vi "Read Arm Pot and Encoder Values.vi"(0 "error in (no error)":errorcluster) -> (1 "armPotValue":dbl, 2 "error out":errorcluster)   [LabVIEW 2019]
uses:
  Global Arm Variables.vi
  <vilib>/Rock Robotics/Network Tables/NT Write Number.vi
  <vilib>/Rock Robotics/Network Tables/NT Write Boolean.vi
panel:
  out "IllegalRangeForExtendedArm":bool
  out "armAngle(degrees)":sgl
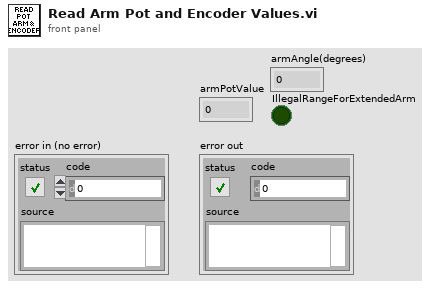
[diagram p1: front panel]
types:
  T1 = typedef "WPI_PotentiometerDevRef.ctl" = cluster{"DevStatus":errorcluster, "Analog Channel":T2, "Invert Output":bool}
  T2 = typedef "FPGA_AIChannel.ctl" = enum8{"AI 0", "AI 1", "AI 2", "AI 3", "AI MXP 0", "AI MXP 1", "AI MXP 2", "AI MXP 3", "Invalid"}
  T3 = typedef "WPI_EncoderDevRef.ctl" = cluster{"DevStatus":errorcluster, "EncoderIndex":T4, "CounterIndex":T5, "DistancePerCount":dbl, "Decoding Type":T6}
  T4 = typedef "FPGA_EncoderIdx.ctl" = enum8{"Enc 0", "Enc 1", "Enc 2", "Enc 3", "Enc 4", "Enc 5", "Enc 6", "Enc 7", "Invalid"}
  T5 = typedef "FPGA_CounterCtrSystemIndex.ctl" = enum8{"Ctr 0", "Ctr 1", "Ctr 2", "Ctr 3", "Ctr 4", "Ctr 5", "Ctr 6", "Ctr 7", "Invalid"}
  T6 = typedef "WPI_EncoderType.ctl" = enum16{"1x", "2x", "4x"}
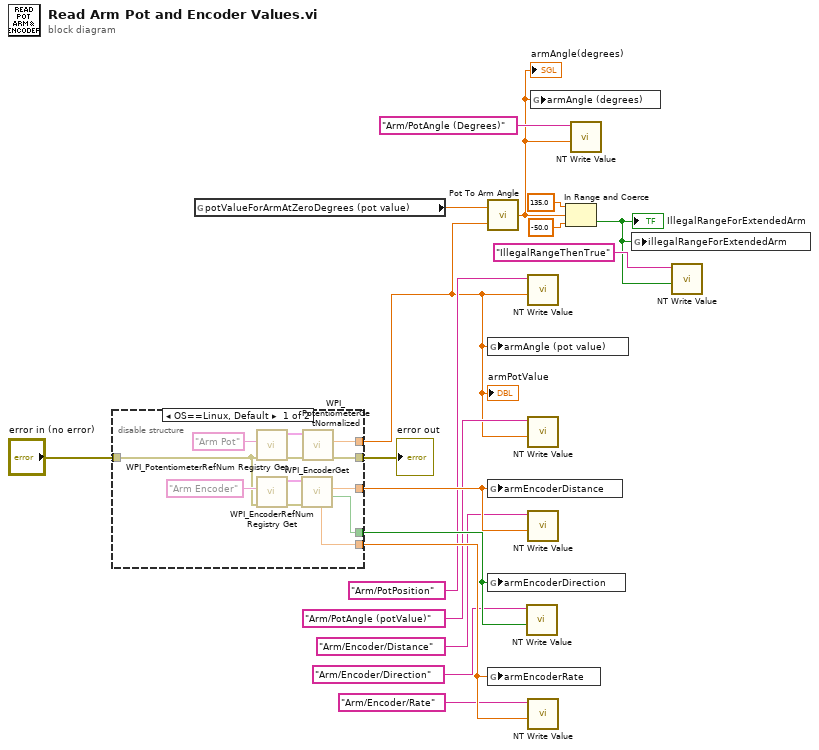
[diagram p0: block diagram]
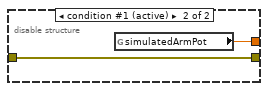
[diagram p2: hidden frame]
diagram:
  n1 = disable-structure shown="OS==Linux, Default" {
    disable-tunnel: "error in (no error)" -> [w24 w32]
    disable-tunnel: [w29 w31] -> w7
    disable-tunnel: [w27 w32] -> w10
    disable-tunnel: [w21 _] -> w17
    disable-tunnel: [w20 _] -> w16
    disable-tunnel: [w19 _] -> w18
    frame condition #0 {
      n2 = call <vilib>:"WPI_PotentiometerRefNum Registry Get.vi"("error in (no error)"=w24, "refnum name"="Arm Pot") -> ("error out"=w28:errorcluster, "PotDevRef"=w30:T1)  [unwired: 8 in]
      n3 = call <vilib>:"WPI_EncoderRefNum Registry Get.vi"("error in (no error)"=w24, "refnum name"="Arm Encoder") -> ("error out"=w23:errorcluster, "EncoderDevRef"=w22:T3)  [unwired: 8 in]
      n4 = call <vilib>:"WPI_EncoderGet.vi"("error in (no error)"=w23, "EncoderDevRef"=w22) -> ("Direction"=w20:bool, "Distance"=w21:dbl, "Rate"=w19:dbl)  [unwired: 4 in, 3 out]
      n5 = call <vilib>:"WPI_PotentiometerGetNormalized.vi"("error in"=w28, "PotDevRef"=w30) -> ("error out"=w27:errorcluster, "Normalized Value"=w29:dbl)  [unwired: 7 in, 1 out]
    }
    frame condition #1 (active) {
      n6 = global read "Global Arm Variables.vi" "simulatedArmPot"() -> (w31:dbl)
    }
  }
  "armPotValue" <- w7
  "error out" <- w10
  n7 = global read "Global Arm Variables.vi" "potValueForArmAtZeroDegrees (pot value)"() -> (w2:dbl)
  n8 = call "Pot To Arm Angle.vi"("simulatedArmPot"=w7, "potValueForArmAtZeroDegrees (pot value)"=w2) -> ("Numeric"=w1:sgl)
  "armAngle(degrees)" <- w1
  n9 = global write "Global Arm Variables.vi" "armAngle (pot value)"(w7) -> ()
  n10 = global write "Global Arm Variables.vi" "armEncoderDistance"(w17) -> ()
  n11 = global write "Global Arm Variables.vi" "armEncoderDirection"(w16) -> ()
  n12 = global write "Global Arm Variables.vi" "armEncoderRate"(w18) -> ()
  n13 = call-poly <vilib>:"NT Write Value.vi"("Boolean"=w16, "Name"="Arm/Encoder/Direction") -> ()  [unwired: 9 in, 1 out]
  n14 = call-poly <vilib>:"NT Write Value.vi"("Numeric"=w7, "Name"="Arm/PotPosition") -> ()  [unwired: 9 in, 1 out]
  n15 = call-poly <vilib>:"NT Write Value.vi"("Numeric"=w7, "Name"="Arm/PotAngle (potValue)") -> ()  [unwired: 9 in, 1 out]
  n16 = call-poly <vilib>:"NT Write Value.vi"("Numeric"=w17, "Name"="Arm/Encoder/Distance") -> ()  [unwired: 9 in, 1 out]
  n17 = call-poly <vilib>:"NT Write Value.vi"("Numeric"=w18, "Name"="Arm/Encoder/Rate") -> ()  [unwired: 9 in, 1 out]
  n18 = global write "Global Arm Variables.vi" "armAngle (degrees)"(w1) -> ()
  n19 = In Range and Coerce(upper limit=sgl 135.0, x=w1, lower limit=sgl -50.0) -> (In Range?=w3:bool)  [unwired: 1 out]
  "IllegalRangeForExtendedArm" <- w3
  n20 = call-poly <vilib>:"NT Write Value.vi"("Numeric"=w1, "Name"="Arm/PotAngle (Degrees)") -> ()  [unwired: 9 in, 1 out]
  n21 = global write "Global Arm Variables.vi" "illegalRangeForExtendedArm"(w3) -> ()
  n22 = call-poly <vilib>:"NT Write Value.vi"("Boolean"=w3, "Name"="IllegalRangeThenTrue") -> ()  [unwired: 9 in, 1 out]
